vi "HV_Status_Main.vi"(11 "Status Array":string[][](array[string])) -> (1 "Rampdown":bool[](array[boolean]), 2 "Rampup":bool[](array[boolean]), 3 "On/Off":bool[](array[boolean]))   [LabVIEW 2019]
panel:
  # "- Monitor status of channels"
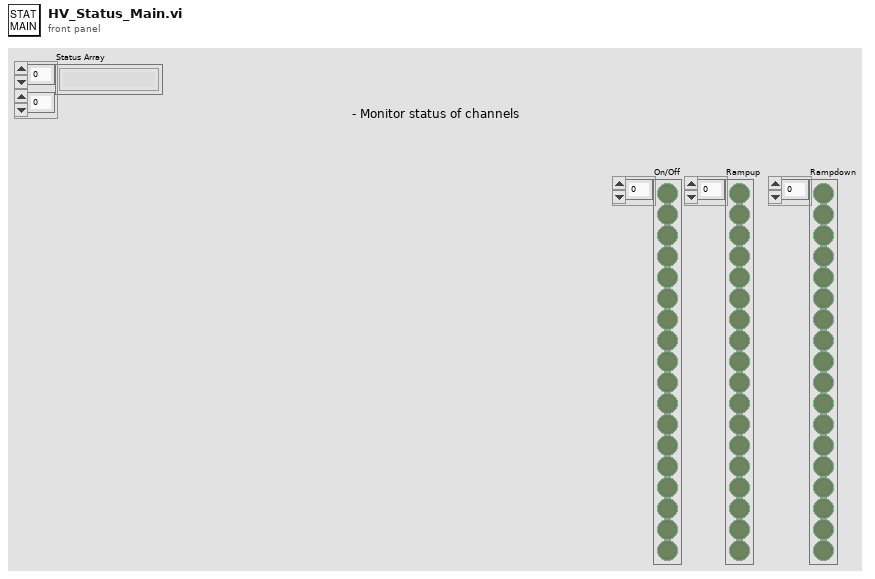
[diagram p1: front panel]
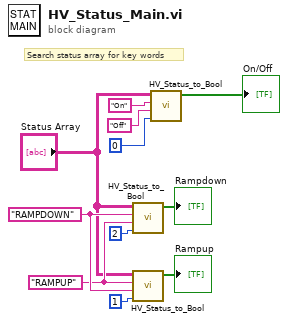
[diagram p0: block diagram]
diagram:
  w9 = "RAMPDOWN" ("false string")
  w8 = "RAMPUP" ("true string")
  # "Search status array for key words"
  n1 = call "HV_Status_to_Bool.vi"("Column"=2, "False"=w8, "True"=w9, "Status Array"="Status Array") -> ("Array"=→"Rampdown":bool[])  [unwired: 7 in]
  n2 = call "HV_Status_to_Bool.vi"("Column"=1, "False"=w9, "True"=w8, "Status Array"="Status Array") -> ("Array"=→"Rampup":bool[])  [unwired: 7 in]
  n3 = call "HV_Status_to_Bool.vi"("Column"=0, "False"="Off" ("false string"), "True"="On" ("true string"), "Status Array"="Status Array") -> ("Array"=→"On/Off":bool[])  [unwired: 7 in]
